vi "FPGA_DMAReadConfig.vi"(8 "error in (no error)":errorcluster, 11 "DMADevRef In":T7) -> (0 "error out":errorcluster, 1 "Enable":T6, 2 "Pause":bool, 3 "DMADevRef Out":T7, 4 "SampleClock":T5)   [LabVIEW 2017]
uses:
  <vilib>/Rock Robotics/SystemInterfaces/DMA/FPGA_DMADevRef.ctl
  <vilib>/Rock Robotics/SystemInterfaces/DMA/FPGA_DMAEnable.ctl
  <vilib>/Rock Robotics/SystemInterfaces/CounterEncoderSourceConvertion/FPGA_CounterEncoderSourceConvertionLVSourceType.ctl
  <vilib>/Rock Robotics/SystemInterfaces/DIO/FPGA_DIODigitalSourceChannel.ctl
  <vilib>/Rock Robotics/SystemInterfaces/AnalogTrigger/FPGA_AnalogTriggerIndex.ctl
  <vilib>/Rock Robotics/SystemInterfaces/AnalogTrigger/FPGA_AnalogTriggerOutType.ctl
  <vilib>/Rock Robotics/SystemInterfaces/System/FPGA_SystemFPGA Ref Global.vi
  <vilib>/Utility/error.llb/Error Cluster From Error Code.vi
  <vilib>/rvi/errors/niLvFpgaAdjustHostInterfaceError.vi
  <vilib>/rvi/interface/nirviReadWriteControl/nirviReadWriteControl.xnode
  <vilib>/Rock Robotics/SystemInterfaces/System/FPGA_SystemFRC FPGA Ref.ctl
  NiFpgaLv.dll
  <vilib>/rvi/interface/Simulation/niFpgaSimulationCallBeginRW.vi
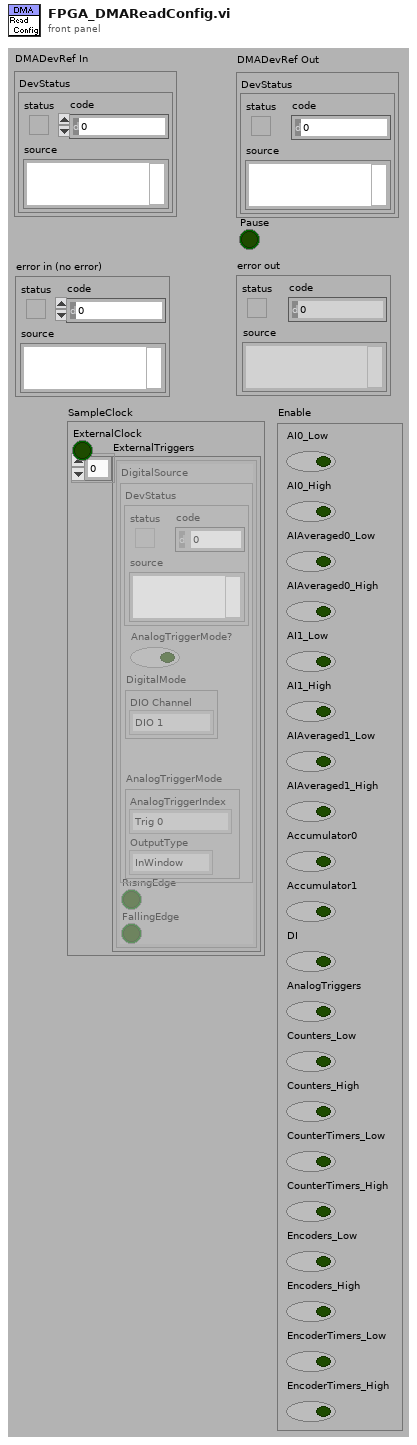
[diagram p1: front panel]
types:
  T1 = typedef "FPGA_CounterEncoderSourceConvertionLVSourceType.ctl" = cluster{"DevStatus":errorcluster, "AnalogTriggerMode?":bool, "DigitalMode":cluster{"DIO Channel":T2}, "AnalogTriggerMode":cluster{"AnalogTriggerIndex":T3, "OutputType":T4}}
  T2 = typedef "FPGA_DIODigitalSourceChannel.ctl" = enum8{"DIO 0", "DIO 1", "DIO 2", "DIO 3", "DIO 4", "DIO 5", "DIO 6", "DIO 7", "DIO 8", "DIO 9", "DIO MXP 0", "DIO MXP 1", "DIO MXP 2", "DIO MXP 3", "DIO MXP 4", "DIO MXP 5", "DIO MXP 6", "DIO MXP 7", "DIO MXP 8", "DIO MXP 9", "DIO MXP 10", "DIO MXP 11", "DIO MXP 12", "DIO MXP 13", "DIO MXP 14", "DIO MXP 15", "Disabled"}
  T3 = typedef "FPGA_AnalogTriggerIndex.ctl" = enum8{"Trig 0", "Trig 1", "Trig 2", "Trig 3", "Trig 4", "Trig 5", "Trig 6", "Trig 7", "Invalid"}
  T4 = typedef "FPGA_AnalogTriggerOutType.ctl" = enum16{"InWindow", "TriggerState", "Rising", "Falling"}
  T5 = cluster{"ExternalClock":bool, "ExternalTriggers":cluster{"DigitalSource":T1, "RisingEdge":bool, "FallingEdge":bool}[]}
  T6 = typedef "FPGA_DMAEnable.ctl" = cluster{"AI0_Low":bool, "AI0_High":bool, "AIAveraged0_Low":bool, "AIAveraged0_High":bool, "AI1_Low":bool, "AI1_High":bool, "AIAveraged1_Low":bool, "AIAveraged1_High":bool, "Accumulator0":bool, "Accumulator1":bool, "DI":bool, "AnalogTriggers":bool, "Counters_Low":bool, "Counters_High":bool, "CounterTimers_Low":bool, "CounterTimers_High":bool, "Encoders_Low":bool, "Encoders_High":bool, "EncoderTimers_Low":bool, "EncoderTimers_High":bool}
  T7 = typedef "FPGA_DMADevRef.ctl" = cluster{"DevStatus":errorcluster}
  T8 = typedef "FPGA_SystemFRC FPGA Ref.ctl" = refnum<k20>
  T9 = cluster{"Pause":bool, "Enable":cluster{"AI0_Low":bool, "AI0_High":bool, "AIAveraged0_Low":bool, "AIAveraged0_High":bool, "AI1_Low":bool, "AI1_High":bool, "AIAveraged1_Low":bool, "AIAveraged1_High":bool, "Accumulator0":bool, "Accumulator1":bool, "DI":bool, "AnalogTriggers":bool, "Counters_Low":bool, "Counters_High":bool, "CounterTimers_Low":bool, "CounterTimers_High":bool, "Encoders_Low":bool, "Encoders_High":bool, "EncoderTimers_Low":bool, "EncoderTimers_High":bool}, "ExternalClock":bool}
  T10 = cluster{"ExternalClockSource":cluster{"Channel":fxp<+,4,4>, "Module":fxp<+,1,1>, "AnalogTrigger":bool}, "RisingEdge":bool, "FallingEdge":bool}[]
  T11 = cluster{"Channel":fxp<+,4,4>, "Module":fxp<+,1,1>, "AnalogTrigger":bool}
  T12 = cluster{"DigitalSource":T1, "RisingEdge":bool, "FallingEdge":bool}
  T13 = cluster{"AI0_Low":bool, "AI0_High":bool, "AIAveraged0_Low":bool, "AIAveraged0_High":bool, "AI1_Low":bool, "AI1_High":bool, "AIAveraged1_Low":bool, "AIAveraged1_High":bool, "Accumulator0":bool, "Accumulator1":bool, "DI":bool, "AnalogTriggers":bool, "Counters_Low":bool, "Counters_High":bool, "CounterTimers_Low":bool, "CounterTimers_High":bool, "Encoders_Low":bool, "Encoders_High":bool, "EncoderTimers_Low":bool, "EncoderTimers_High":bool}
  T14 = cluster{"ExternalClock":bool, cluster{"DigitalSource":T1, "RisingEdge":bool, "FallingEdge":bool}[]}
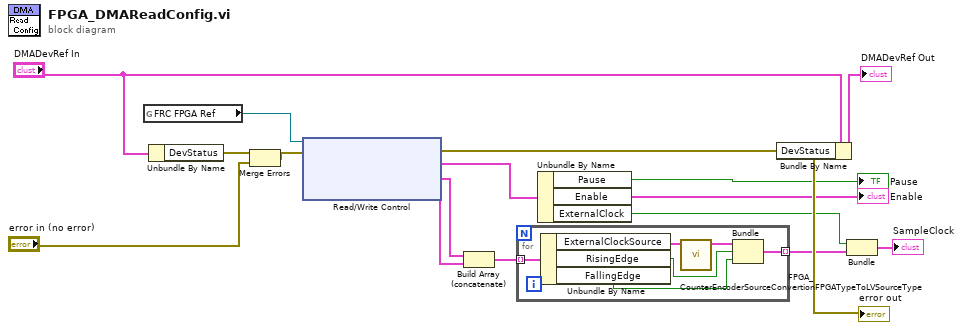
[diagram p0: block diagram]
diagram:
  n1 = global read "FPGA_SystemFPGA Ref Global.vi" "FRC FPGA Ref"() -> (w5:T8)
  n2 = Unbundle By Name("DMADevRef In") -> ("DevStatus"=w3:errorcluster)
  n3 = Merge Errors(w3, "error in (no error)") -> (w4:errorcluster)
  n4 = xnode "Read/Write Control"("FPGA VI Reference In"=w5, "error in"=w4) -> ("error out"=w13:errorcluster, "DMA.Config"=w7:T9, "DMA.ExternalTriggers0"=w6:T10, "DMA.ExternalTriggers1"=w1:T10)  [unwired: 1 out]
  "error out" <- w13
  n5 = Build Array (concatenate)(w6, w1) -> (w2:T10)
  n6 = for {
    tunnel: [w17] -> w9 mode=indexing
    tunnel: w2 -> [w22] mode=indexing
    n7 = Unbundle By Name(w22) -> ("ExternalClockSource"=w21:T11, "RisingEdge"=w19:bool, "FallingEdge"=w18:bool)
    n8 = call <vilib>:"FPGA_CounterEncoderSourceConvertionFPGATypeToLVSourceType.vi"("FPGASource"=w21) -> ("DigitalSource"=w20:T1)  [unwired: 10 out]
    n9 = Bundle("DigitalSource"=w20, "RisingEdge"=w19, "FallingEdge"=w18) -> (w17:T12)  [unwired: 1 out]
  }
  n10 = Unbundle By Name(w7) -> ("Pause"=→"Pause":bool, "Enable"=→"Enable":T13, "ExternalClock"=w10:bool)
  n11 = Bundle By Name(cluster="DMADevRef In", "DevStatus"=w13) -> (→"DMADevRef Out":T7)
  n12 = Bundle("ExternalClock"=w10, w9) -> (→"SampleClock":T14)  [unwired: 1 out]
